vi "RPM Testing.vi"() -> (3 "interpolation value":dbl format="%0.2f")   [LabVIEW 2019]
uses:
  <vilib>/Analysis/NI_AALPro.lvlib
  2021 Team Code/Robot Global Data.vi
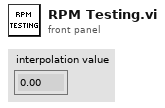
[diagram p1: front panel]
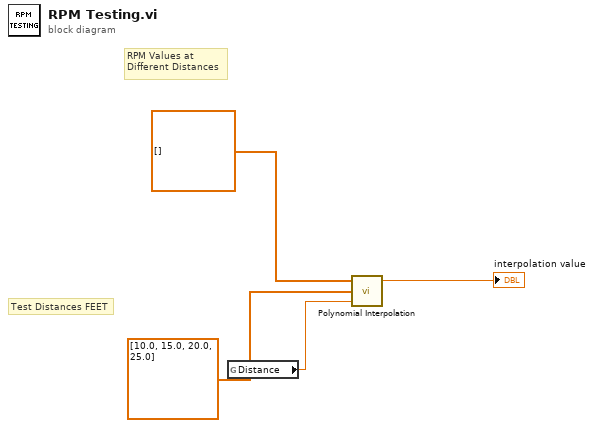
[diagram p0: block diagram]
diagram:
  # "Test Distances FEET"
  # "RPM Values at\nDifferent Distances"
  n1 = global read "Robot Global Data.vi" "Distance"() -> (w2:dbl)
  n2 = call <vilib>:"Polynomial Interpolation.vi"("x value"=w2, "X"=dbl[] [10.0, 15.0, 20.0, 25.0], "Y"=dbl[] []) -> ("interpolation value"=→"interpolation value":dbl)  [unwired: 2 out]
